vi "Load actor from configuration.vi"(8 "error in (no error)":errorcluster, 9 "Type":string, 10 "Configuration":T2, 11 "Registry":T1) -> (0 "error out":errorcluster, 3 "Actor":refnum<class "Actor.lvclass">)   [LabVIEW 2014]
uses:
  Configuration.ctl
  Registry.ctl
  <vilib>/ActorFramework/Actor/Actor.lvclass
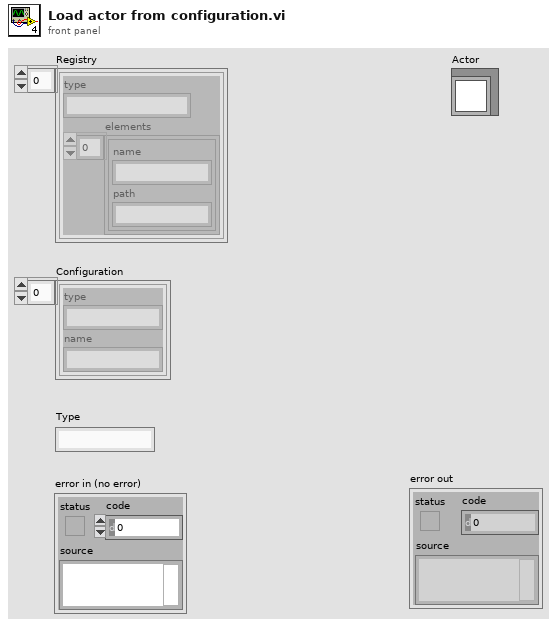
[diagram p1: front panel]
types:
  T1 = typedef "Registry.ctl" = cluster{"type":string, "elements":cluster{"name":string, "path":string}[]}[]
  T2 = typedef "Configuration.ctl" = cluster{"type":string, "name":string}[]
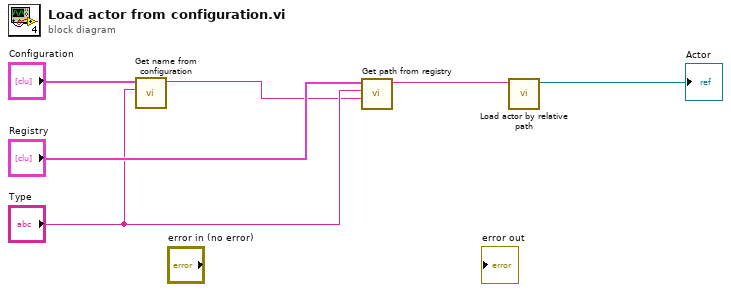
[diagram p0: block diagram]
diagram:
  n1 = call "Get name from configuration.vi"("Configuration"="Configuration", "Type"="Type") -> ("Name"=w1:string)  [unwired: 7 in, 1 out]
  n2 = call "Get path from registry.vi"("Name"=w1, "Type"="Type", "Registry"="Registry") -> ("Path"=w4:string)  [unwired: 7 in, 1 out]
  n3 = call "Load actor by relative path.vi"("Path"=w4) -> ("Actor"=→"Actor":refnum<class "Actor.lvclass">)  [unwired: 9 in, 1 out]
